vi "ExSpectralCalCollectStore.vi"() -> ()   [LabVIEW 2010]
panel:
  in  "Path":path
  out "XY Graph":T1(graph)
  in  "Pixel Width (microns)":dbl=25.0 format="%.2f"
  in  "Magnification":dbl=1.0 format="%.2f"
  in  "Detector Angle (degrees)":dbl=1.0 format="%.2f"
  in  "Inclusion Angle (degrees)":dbl=1.0 format="%.2f"
  in  "Focal Length (mm)":dbl=300.0 format="%.2f"
  in  "Slope Adjust":dbl format="%.2f"
  in  "Center Offset":dbl format="%.2f"
  in  "Start Wavelength":dbl format="%.2f"
  in  "Grating Speed":dbl=2000.0 min=1.0 step=1.0 format="%.2f"
  in  "Grating number":i16=1 min=1 max=100 step=1
  in  "Temperature":dbl=-10.0 format="%.2f"
  in  "Exposure":dbl min=0.0 step=0.001 format="%.3f"
  out "error out":errorcluster
  in  "error in (no error)":errorcluster
  # "ExSpectralCalCollectStore.vi\n(Normal Spectrograph via \nUSB/COM port)\nNote that appropriate calibration\ninformation for the spectrometer\nmust be entered before running.\nCamera and Spectrometer control.  This vi will open both the camera and spectrograph.  It will then move the grating to the Start Wavelength.  Data will then be collected and displayed. The data and the display will be calibrated from information generated from spectrometer and input information to the left."
  # "NOTES:\nIf required, a properly configured camera .ini file must be present for camera operation.\n\nThe properly configured spectrometer .ini file must be present in the LabVIEW folder for spectrograph operation.\n\nConsult the documentation for more information on how to configure these files."
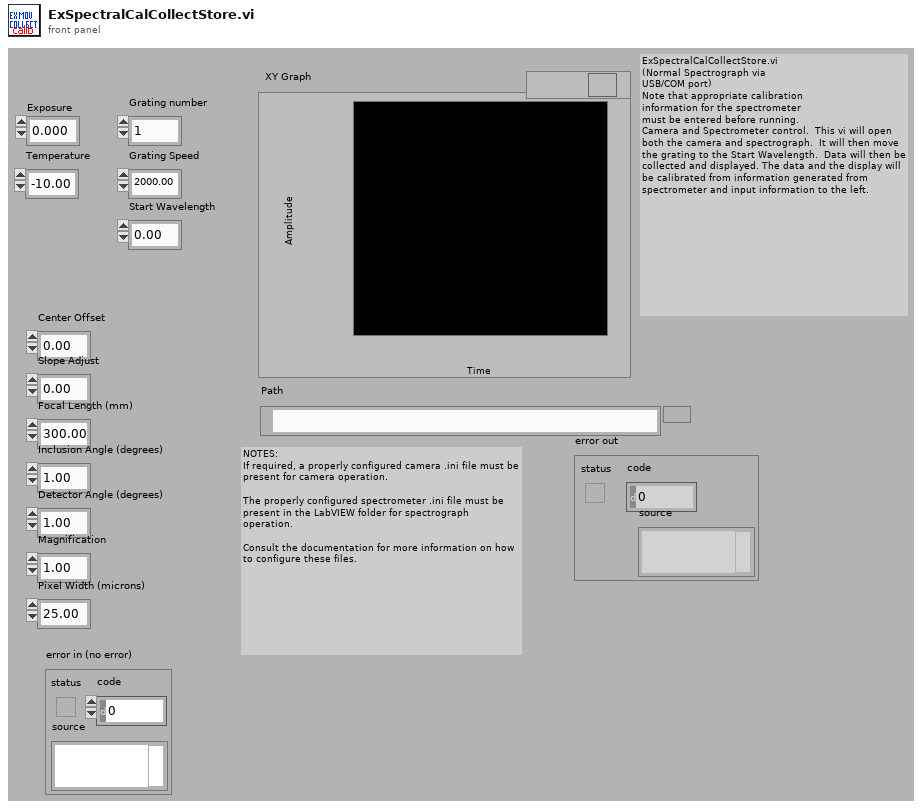
[diagram p1: front panel]
types:
  T1 = cluster{"Calibrated Array":dbl[], "Array F32":sgl[]}
  T2 = cluster{"Center Offset":dbl, "Slope Adjust":dbl, "Focal Length (mm)":dbl, "Inclusion Angle (degrees)":dbl, "Detector Angle (degrees)":dbl, "Magnification":dbl, "Pixel Width (microns)":dbl}
  T3 = cluster{"Camera Handle":u32, "Pulser Handle":u32, "File Handle":u32, "Display Handle":u32, "Image Handle":u32}
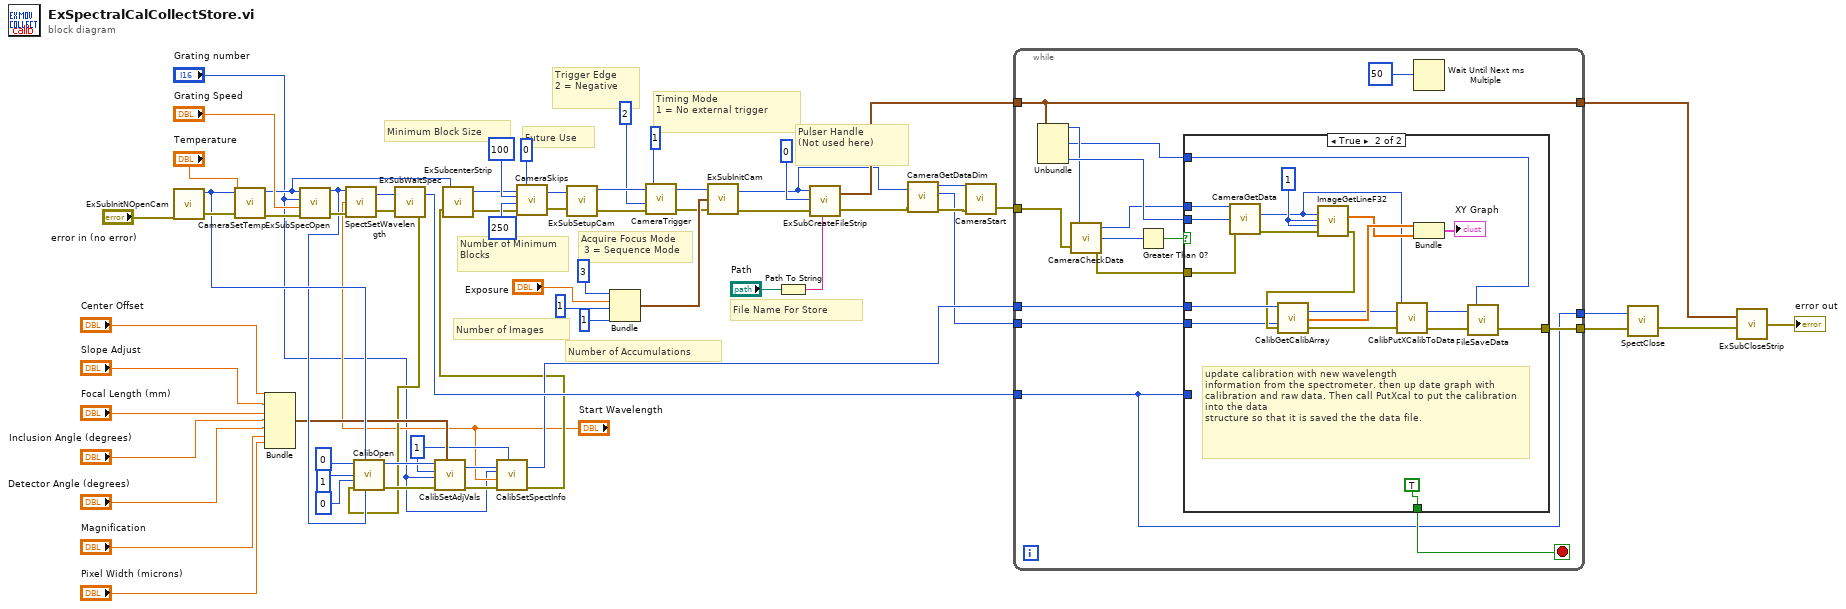
[diagram p0: block diagram]
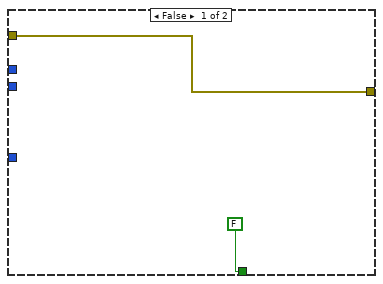
[diagram p2: hidden frame]
diagram:
  w15 = 1
  # "Pulser Handle\n(Not used here)"
  # "Trigger Edge\n2 = Negative"
  # "Timing Mode\n1 = No external trigger"
  # "Future Use"
  # "Number of Minimum Blocks"
  # "Minimum Block Size"
  # "Number of Images"
  # "Number of Accumulations"
  # "Acquire Focus Mode\n 3 = Sequence Mode"
  # "File Name For Store"
  n1 = call "ExSubInitNOpenCam.vi"("error in (no error)"="error in (no error)") -> ("Camera Handle"=w29:u32, "error out"=w33:errorcluster)
  n2 = call <userlib>:"CameraSetTemp.vi"("error in (no error)"=w33, "Temperature"="Temperature", "Camera Handle"=w29) -> ("error out"=w34:errorcluster, "Camera Handle"=w26:u32)
  n3 = Bundle("Center Offset"="Center Offset", "Slope Adjust"="Slope Adjust", "Focal Length (mm)"="Focal Length (mm)", "Inclusion Angle (degrees)"="Inclusion Angle (degrees)", "Detector Angle (degrees)"="Detector Angle (degrees)", "Magnification"="Magnification", "Pixel Width (microns)"="Pixel Width (microns)") -> (w18:T2)  [unwired: 1 in]
  n4 = call "ExSubSpecOpen.vi"("error in (no error)"=w34, "Grating speed"="Grating Speed", "Grating number"="Grating number", "Camera Handles"=w26) -> ("error out"=w38:errorcluster, "Spectrometer Handle"=w27:u32)  [unwired: 1 out]
  n5 = call <userlib>:"SpectSetWavelength.vi"("error in"=w38, "Wavelength"="Start Wavelength", "Spectrometer Handle"=w27) -> ("error out"=w41:errorcluster, "Spectrumeter Handle"=w40:u32)
  n6 = call "ExSubWaitSpec.vi"("error in (no error)"=w41, "Spectrometer Handle"=w40) -> ("error out"=w14:errorcluster, "Spectrometer handle"=w39:u32)
  n7 = call <userlib>:"CalibOpen.vi"("Spectrometer Handle"=w27, "Detector Handle"=w29, "error in"=w14, "Detector Position"=0, "Calibration Type"=1, "Calibration Device ID"=0) -> ("error out"=w16:errorcluster, "Calibration Handle"=w17:u32)
  n8 = call <userlib>:"CalibSetAdjVals.vi"("Calibration Handle"=w17, "Turret Number"=w15, "Grating Number"="Grating number", "error in"=w16, "Spectrometer Calibration Parameters"=w18) -> ("Calibration Handle"=w12:u32, "error out"=w10:errorcluster)
  n9 = call <userlib>:"CalibSetSpectInfo.vi"("Calibration Handle"=w12, "Current Grating Number"="Grating number", "Current Wavelength"="Start Wavelength", "error in"=w10, "Current Turret Number"=w15) -> ("Calibration Handle"=w13:u32, "error out"=w11:errorcluster)
  n10 = call "ExSubcenterStrip.vi"("error in (no error)"=w11, "Camera Handle"=w26) -> ("error out"=w43:errorcluster, "Camera Handle"=w44:u32)
  n11 = call <userlib>:"CameraSkips.vi"("Camera Handle"=w44, "Minimum Block Size"=100, "Number of Minimum blocks"=250, "error in"=w43, "Type of Skips"=0) -> ("Camera Handle"=w46:u32, "error out"=w45:errorcluster)
  n12 = call "ExSubSetupCam.vi"("error in (no error)"=w45, "Camera Handle"=w46) -> ("error out"=w51:errorcluster, "Camera Handle"=w55:u32)
  n13 = Bundle(3, "Exposure"="Exposure", 1, 1) -> (w62:cluster{i32, "Exposure":dbl, i32, i32})  [unwired: 1 in]
  n14 = call <userlib>:"CameraTrigger.vi"("error in"=w51, "Trigger Edge"=2, "Timing Mode"=1, "Camera Handle"=w55) -> ("error out"=w56:errorcluster, "Camera Handle"=w54:u32)
  n15 = call "ExSubInitCam.vi"("error in (no error)"=w56, "Camera Information"=w62, "Camera Handle"=w54) -> ("error out"=w61:errorcluster, "Camera Handle"=w8:u32)
  n16 = Path To String(path="Path") -> (string=w2:string)
  n17 = call "ExSubCreateFileStrip.vi"("error in (no error)"=w61, "File and Display Name"=w2, "Pulser Handle"=0, "Camera Handle"=w8) -> ("error out"=w4:errorcluster, "Handles Out"=w59:T3)
  n18 = call <userlib>:"CameraGetDataDim.vi"("Camera Handle"=w8, "error in"=w4) -> ("Camera Handle"=w7:u32, "Xdim"=w5:u32, "error out"=w6:errorcluster)  [unwired: 1 out]
  n19 = call <userlib>:"CameraStart.vi"("error in"=w6, "Camera Handle"=w7) -> ("error out"=w47:errorcluster)  [unwired: 1 out]
  n20 = while {
    tunnel: w59 -> [w81]
    tunnel: w47 -> [w80]
    tunnel: [w78] -> w35
    tunnel: [w81] -> w58
    tunnel: w39 -> [w68]
    tunnel: [w68] -> w36
    tunnel: w13 -> [w72]
    tunnel: w5 -> [w70]
    stop <- w71 stop-if-true
    n21 = Unbundle(w81) -> ("Camera Handle"=w76:u32, "File Handle"=w69:u32, "Image Handle"=w77:u32)  [unwired: 2 out]
    n22 = call <userlib>:"CameraCheckData.vi"("Camera Handle"=w76, "error in"=w80) -> ("Camera Handle"=w75:u32, "Number Of Frames Available"=w73:i32, "error out"=w79:errorcluster)
    n23 = Greater Than 0?(x=w73) -> (x > 0?=w74:bool)
    n24 = case shown="True" w74 {
      tunnel: w79 -> [w84 w103]
      tunnel: [w84 w87] -> w78
      tunnel: w77 -> [_ w101]
      tunnel: w75 -> [_ w100]
      tunnel: w68 -> [_ _]
      tunnel: w72 -> [_ w94]
      tunnel: [FALSE TRUE] -> w71
      tunnel: w70 -> [_ w92]
      tunnel: w69 -> [_ w85]
      frame False {
      }
      frame True {
        w102 = 1
        # "update calibration with new wavelength\ninformation from the spectrometer. then up date graph with calibration and raw data. Then call PutXcal to put the calibration into the data\nstructure so that it is saved the the data file."
        n25 = call <userlib>:"CameraGetData.vi"("error in"=w103, "Data Handle"=w101, "Camera Handle"=w100) -> ("error out"=w99:errorcluster, "Data Handle"=w91:u32)  [unwired: 1 out]
        n26 = call <userlib>:"ImageGetLineF32.vi"("error in"=w99, "Z Position"=w102, "Y Position"=w102, "Data Handle"=w91) -> ("error out"=w93:errorcluster, "Array F32"=w97:sgl[])  [unwired: 1 out]
        n27 = call <userlib>:"CalibGetCalibArray.vi"("error in"=w93, "Array Size"=w92, "Calibration Handle"=w94) -> ("error out"=w89:errorcluster, "Calibrated Array"=w98:dbl[], "Calibration Handle"=w90:u32)
        n28 = call <userlib>:"CalibPutXCalibToData.vi"("error in (no error)"=w89, "Calibration Handle"=w90, "Data Handle"=w91) -> ("error out"=w88:errorcluster, "Data Handle"=w86:u32)
        n29 = Bundle("Calibrated Array"=w98, "Array F32"=w97) -> (→"XY Graph":T1)  [unwired: 1 in]
        n30 = call <userlib>:"FileSaveData.vi"("error in"=w88, "Image Handle"=w86, "File Handle"=w85) -> ("error out"=w87:errorcluster)  [unwired: 1 out]
      }
    }
    n31 = Wait Until Next ms Multiple(millisecond multiple=50) -> ()  [unwired: 1 out]
  }
  n32 = call <userlib>:"SpectClose.vi"("error in"=w35, "Spectrometer Handle"=w36) -> ("error out"=w37:errorcluster)
  n33 = call "ExSubCloseStrip.vi"("error in (no error)"=w37, "Handles In"=w58) -> ("error out"=→"error out":errorcluster)
